vi "PCSMain.contents.vi"   [LabVIEW 2014, in "PCSMain.lvlib"]
doc: "This class is forseen to select PHELIX devices to work with. Therefore it reads the data base. It also opens a connection to other PCS nodes.\n\nThis class is part of the PHELIX user layer."
uses:
  PCSMain.lvlib
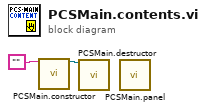
[diagram p0: block diagram]
diagram:
  n1 = call "PCSMain.constructor.vi"("name"="") -> ("i ref out"=w1:refnum<vi>)  [unwired: 16 in, 2 out]
  n2 = call "PCSMain.destructor.vi"("i ref in"=w1) -> ()  [unwired: 18 in, 1 out]
  n3 = call "PCSMain.panel.vi"() -> ()  [unwired: 19 in, 1 out]
